vi "Add.vi"() -> ()   [LabVIEW 2020, in "Basic_Operations.lvlib"]
uses:
  Basic_Operations.lvlib
  <vilib>/Wiresmith Technology/G CLI/CLI Class/CLI.lvclass
panel:
  out "Sum Result":dbl
  in  "B":dbl=20.0
  in  "A":dbl=10.0
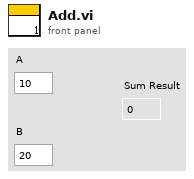
[diagram p1: front panel]
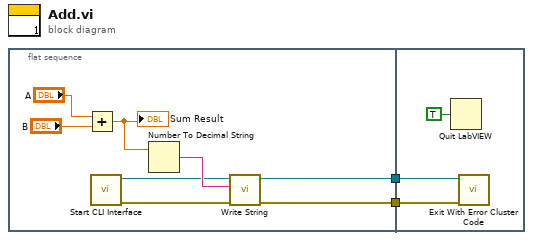
[diagram p0: block diagram]
diagram:
  n1 = flat-sequence {
    tunnel: [w4] -> w2
    tunnel: [w3] -> w1
    tunnel: w2 -> [w12]
    tunnel: w1 -> [w11]
    frame #0 {
      n2 = Add(x="A", y="B") -> (x+y=w8:dbl)
      "Sum Result" <- w8
      n3 = call <vilib>:"Start CLI Interface.vi"() -> ("error out"=w5:errorcluster, "CLI out"=w6:refnum<class "CLI.lvclass">)  [unwired: 8 in, 2 out]
      n4 = Number To Decimal String(number=w8) -> (decimal integer string=w7:string)  [unwired: 1 in]
      n5 = call <vilib>:"Write String.vi"("error in (no error)"=w5, "Text to Write"=w7, "CLI in"=w6) -> ("error out"=w3:errorcluster, "CLI out"=w4:refnum<class "CLI.lvclass">)  [unwired: 7 in]
    }
    frame #1 {
      n6 = Quit LabVIEW(quit? (T)=TRUE) -> ()
      n7 = call <vilib>:"Exit With Error Cluster Code.vi"("error in (no error)"=w11, "CLI in"=w12) -> ()  [unwired: 9 in, 1 out]
    }
  }
